vi "LVH5Rget_obj_type.vi"   [LabVIEW 2017]
doc: "Retrieves the type of object that an object reference points to."
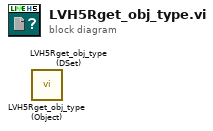
[diagram p0: block diagram]
diagram:
  n1 = call <vilib>:"LVH5Rget_obj_type (Object).vi"() -> ()  [unwired: 7 in, 3 out]
  n2 = call <vilib>:"LVH5Rget_obj_type (DSet).vi"() -> ()  [unwired: 7 in, 3 out]
